vi "Sum_Erros.vi"(11 "array error status":T1[](array[typedef])) -> (3 "Alarms":T2)   [LabVIEW 2018]
uses:
  Controls/Clusts/DigOutClust.ctl
  Controls/Clusts/ErrorStatus.ctl
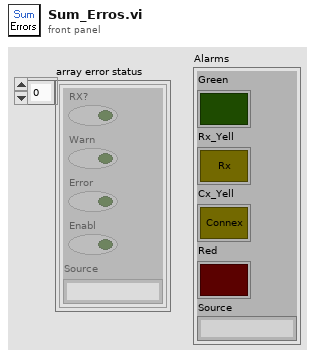
[diagram p1: front panel]
types:
  T1 = typedef "ErrorStatus.ctl" = cluster{"RX?":bool, "Warn":bool, "Error":bool, "Enabl":bool, "Source":string}
  T2 = typedef "DigOutClust.ctl" = cluster{"Green":bool, "Rx_Yell":bool, "Cx_Yell":bool, "Red":bool, "Source":string}
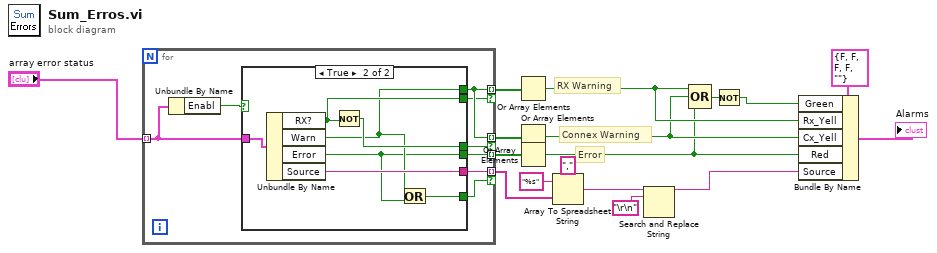
[diagram p0: block diagram]
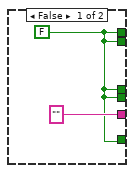
[diagram p2: hidden frame]
diagram:
  # "Error"
  # "Connex Warning"
  # "RX Warning"
  n1 = for {
    tunnel: "array error status" -> [w21] mode=indexing
    tunnel: [w25] -> w15 mode=indexing if=w22
    tunnel: [w25] -> w16 mode=indexing if=w23
    tunnel: [w24] -> w17 mode=indexing
    tunnel: [w19] -> w6 mode=indexing if=w18
    n2 = Unbundle By Name(w21) -> ("Enabl"=w20:bool)
    n3 = case shown="True" w20 {
      tunnel: [w26 w30] -> w25
      tunnel: [w26 w29] -> w24
      tunnel: [w26 w34] -> w23
      tunnel: [w26 w33] -> w22
      tunnel: w21 -> [_ w32]
      tunnel: ["" ("Source") w31] -> w19
      tunnel: [w26 w28] -> w18
      frame False {
        w26 = FALSE ("Warn")
      }
      frame True {
        n4 = Unbundle By Name(w32) -> ("RX?"=w33:bool, "Warn"=w30:bool, "Error"=w29:bool, "Source"=w31:string)
        n5 = Not(x=w33) -> (.not. x?=w34:bool)
        n6 = Or(x=w30, y=w29) -> (x .or. y?=w28:bool)
      }
    }
  }
  n7 = Or Array Elements(Boolean array=w15) -> (logical OR=w13:bool)
  n8 = Or Array Elements(Boolean array=w16) -> (logical OR=w12:bool)
  n9 = Or Array Elements(Boolean array=w17) -> (logical OR=w11:bool)
  n10 = Array To Spreadsheet String(delimiter (Tab)=",", array=w6, 3:"%s" ("format string")) -> (spreadsheet string=w2:string)
  n11 = Search and Replace String(input string=w2, search string="\r\n") -> (result string=w1:string)  [unwired: 6 in, 3 out]
  n12 = Compound Arithmetic op=OR(w13, w12, w11) -> (w9:bool)
  n13 = Not(x=w9) -> (.not. x?=w10:bool)
  n14 = Bundle By Name(cluster=T2 {"Green"=FALSE, "Rx_Yell"=FALSE, "Cx_Yell"=FALSE, "Red"=FALSE, "Source"=""} ("Alarms 2"), "Green"=w10, "Rx_Yell"=w13, "Cx_Yell"=w12, "Red"=w11, "Source"=w1) -> (→"Alarms":T2)
